vi "Merge Configs.vi"(7 "Dispose From Config (T)":bool=TRUE, 8 "error in (no error)":errorcluster, 9 "Merge Hierarchy (Root)":string[](array[string]), 10 "From Config":refnum<class "Config Manager.lvclass">, 11 "Config Manager in":refnum<class "Config Manager.lvclass">) -> (0 "error out":errorcluster, 3 "Config Manager out":refnum<class "Config Manager.lvclass">)   [LabVIEW 2023, in "CDM-Config.lvlib" / "Config Manager.lvclass"]
doc: "Merges the <b>From</b> Config into this Config. Any elements that are present in <b>From</b> and not in this config will be created, any values that are not blank in <b>From</b> will be written to this config, and Meta fields will be written to this config.\n\nBy default the <b>From</b> config will be cleaned up once the merge completes, leaving it unavailable for further use. To leave it available ensure setting <b>Dispose From Config</b> to False.\n\nOptionally a <b>Merge Hierarchy</b> can be specified and all elements in the <b>From</b> config will be merged in with the specified hierarchy element as the parent."
uses:
  Config Manager.lvclass
  Config Manager.lvclass/Config Manager.ctl
  Config Element/Write Variant Value.vi
  Config Element/Config Element.lvclass
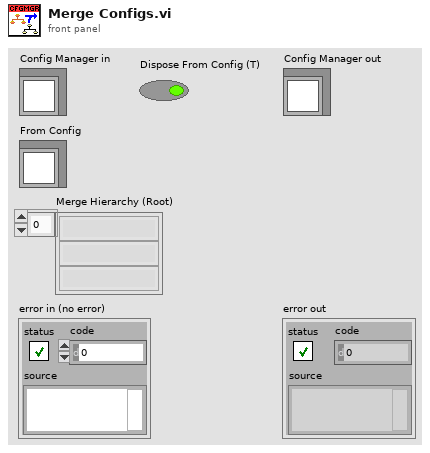
[diagram p1: front panel]
types:
  T1 = typedef "CDM-Config.lvlib/Config Manager.lvclass/Ref Data.ctl" = cluster{"Elements":refnum<class "Config Element.lvclass">[], "Hierarchy Map":map{string[], i32}, "Element Map":map{refnum<class "Config Element.lvclass">, i32}}
  T2 = typedef "CDM-Config.lvlib/Meta Data.ctl" = cluster{"Name":string, "Value":string}
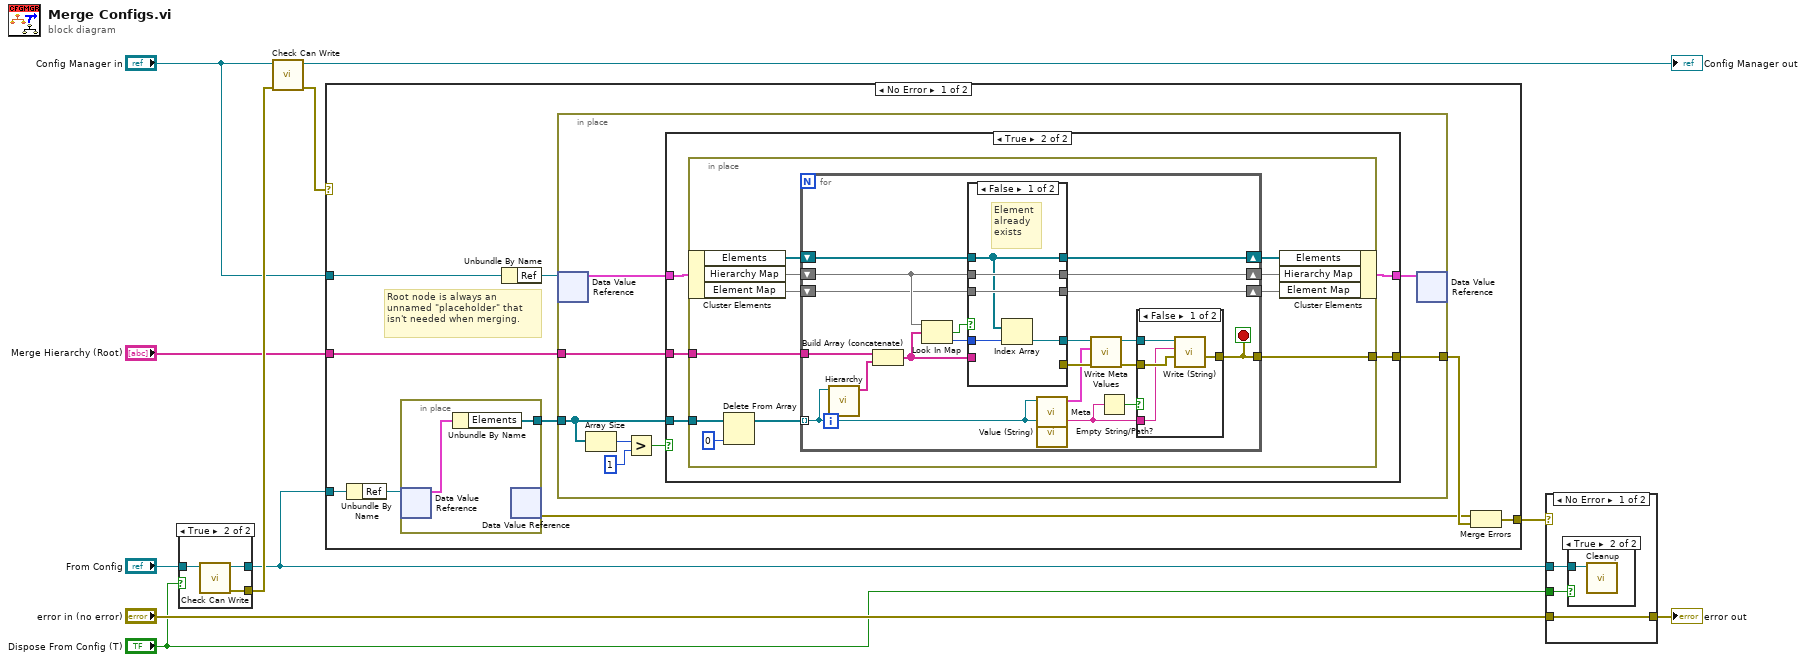
[diagram p0: block diagram]
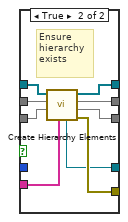
[diagram p3: hidden frame]
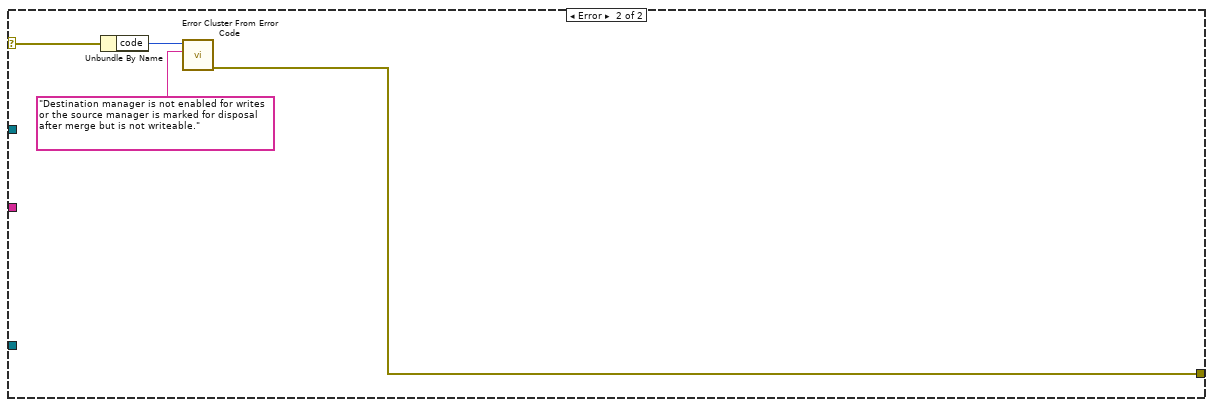
[diagram p5: hidden frame]
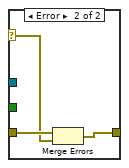
[diagram p8: hidden frame]
diagram:
  n1 = case shown="True" "Dispose From Config (T)" {
    tunnel: "From Config" -> [w12 w15]
    tunnel: [w12 w14] -> w5
    tunnel: [_ w13] -> w11
    frame False {
    }
    frame True {
      n2 = call "Check Can Write.vi"("Config Manager in"=w15) -> ("error out"=w13:errorcluster, "Config Manager out"=w14:refnum<class "Config Manager.lvclass">)  [unwired: 9 in]
    }
  }
  n3 = call "Check Can Write.vi"("error in (no error)"=w11, "Config Manager in"="Config Manager in") -> ("error out"=w1:errorcluster, "Config Manager out"=→"Config Manager out":refnum<class "Config Manager.lvclass">)  [unwired: 8 in]
  n4 = case shown="No Error" w1 {
    selector: w1 -> [_ w94]
    tunnel: [w23 w91] -> w9
    tunnel: "Merge Hierarchy (Root)" -> [w21 _]
    tunnel: w5 -> [w17 _]
    tunnel: "Config Manager in" -> [w16 _]
    frame No Error {
      # "Root node is always an unnamed \"placeholder\" that isn't needed when merging."
      n5 = Unbundle By Name(w17) -> ("Ref"=w20:refnum<data-value>)
      n6 = in-place {
        in-place-border: [w25] -> w19
        n7 = in-place-dvr #1(w20) -> (w26:T1)  [unwired: 1 out]
        n8 = Unbundle By Name(w26) -> ("Elements"=w25:refnum<class "Config Element.lvclass">[])
        n9 = in-place-dvr #1() -> (w18:errorcluster)  [unwired: 1 in, 1 out]
      }
      n10 = Unbundle By Name(w16) -> ("Ref"=w24:refnum<data-value>)
      n11 = in-place {
        in-place-border: [w29] -> w22
        in-place-border: w21 -> [w28]
        in-place-border: w19 -> [w27]
        n12 = in-place-dvr #2(w24) -> (w34:T1)  [unwired: 1 out]
        n13 = Array Size(array=w27) -> (size(s)=w33:i32)
        n14 = Greater?(x=w33, y=1) -> (0:w31:bool)
        n15 = case shown="True" w31 {
          tunnel: w34 -> [w35 w39]
          tunnel: w27 -> [_ w40]
          tunnel: [w35 w38] -> w30
          tunnel: [_ w37] -> w29
          tunnel: w28 -> [_ w36]
          frame False {
            # "From is empty (only has empty root node) so nothing to do."
          }
          frame True {
            n16 = in-place {
              in-place-border: w40 -> [w51]
              in-place-border: [w42] -> w37
              in-place-border: w36 -> [w41]
              n17 = in-place-cluster #3(w39) -> ("Elements"=w48:refnum<class "Config Element.lvclass">[], "Hierarchy Map"=w47:map{string[], i32}, "Element Map"=w46:map{refnum<class "Config Element.lvclass">, i32})
              n18 = Delete From Array(array=w51, index=0) -> (array with subset deleted=w49:refnum<class "Config Element.lvclass">[])  [unwired: 1 in, 1 out]
              n19 = for {
                tunnel: w49 -> [w56] mode=indexing
                shift-right: [w65] -> w43
                shift-left: w46 -> [w68]
                shift-right: [w63] -> w45
                shift-left: w48 -> [w70]
                shift-right: [w64] -> w44
                shift-left: w47 -> [w69]
                tunnel: [w52] -> w42
                tunnel: w41 -> [w60]
                stop <- w52 stop-if-true
                n20 = call "Hierarchy.vi"("Config Element in"=w56) -> ("Hierarchy"=w62:string[])  [unwired: 9 in, 1 out]
                n21 = Build Array (concatenate)(w60, w62) -> (w61:string[])
                n22 = Look In Map(map=w69, key=w61) -> (key not found?=w67:bool, value=w66:i32)  [unwired: 1 in]
                n23 = case shown="False" w67 {
                  tunnel: w70 -> [w73 w85]
                  tunnel: w69 -> [w74 w84]
                  tunnel: w68 -> [w75 w83]
                  tunnel: w66 -> [w76 _]
                  tunnel: [w75 w82] -> w65
                  tunnel: [w74 w81] -> w64
                  tunnel: [w73 w80] -> w63
                  tunnel: w61 -> [_ w79]
                  tunnel: [w72 w77] -> w57
                  tunnel: [_ w78] -> w71
                  frame False {
                    # "Element already exists"
                    n24 = Index Array(array=w73, index=w76) -> (element=w72:refnum<class "Config Element.lvclass">)
                  }
                  frame True {
                    # "Ensure hierarchy exists"
                    n25 = call "Create Hierarchy Elements.vi"("Hierarchy"=w79, "Element Map in"=w83, "Hierarchy Map in"=w84, "Elements in"=w85) -> ("error out"=w78:errorcluster, "Element Map"=w82:map{refnum<class "Config Element.lvclass">, i32}, "Hierarchy Map"=w81:map{string[], i32}, "Elements"=w80:refnum<class "Config Element.lvclass">[], "New Element"=w77:refnum<class "Config Element.lvclass">)  [unwired: 3 in]
                  }
                }
                n26 = call "Meta.vi"("Config Element in"=w56) -> ("Meta Data"=w55:T2[])  [unwired: 9 in, 1 out]
                n27 = call "Value (String).vi"("Config Element in"=w56) -> ("String Value"=w54:string)  [unwired: 9 in, 1 out]
                n28 = call "Write Meta Values.vi"("error in (no error)"=w71, "Meta Data"=w55, "Config Element in"=w57) -> ("error out"=w59:errorcluster, "Config Element out"=w58:refnum<class "Config Element.lvclass">)  [unwired: 7 in]
                n29 = Empty String/Path?(string/path=w54) -> (empty?=w53:bool)
                n30 = case shown="False" w53 {
                  tunnel: [w89 w90] -> w52
                  tunnel: w59 -> [w88 w90]
                  tunnel: w58 -> [w87 _]
                  tunnel: w54 -> [w86 _]
                  frame False {
                    n31 = call "Write (String).vi"("error in (no error)"=w88, "String Value"=w86, "Config Element in"=w87) -> ("error out"=w89:errorcluster)  [unwired: 7 in, 1 out]
                  }
                  frame True {
                  }
                }
              }
              n32 = in-place-cluster #3("Elements"=w45, "Hierarchy Map"=w44, "Element Map"=w43) -> (w38:T1)
            }
          }
        }
        n33 = in-place-dvr #2(w30) -> ()  [unwired: 2 out]
      }
      n34 = Merge Errors(w18, w22) -> (w23:errorcluster)
    }
    frame Error {
      n35 = Unbundle By Name(w94) -> ("code"=w93:i32)
      n36 = call <vilib>:"Error Cluster From Error Code.vi"("error message (\"\")"="Destination manager is not enabled for writes or the source manager is marked for disposal after merge but is not writeable." ("error message (\"\")"), "error code (0)"=w93) -> ("error out"=w91:errorcluster)  [unwired: 7 in]
    }
  }
  n37 = case shown="No Error" w9 {
    selector: w9 -> [_ w100]
    tunnel: w5 -> [w97 _]
    tunnel: "Dispose From Config (T)" -> [w96 _]
    tunnel: "error in (no error)" -> [w95 w101]
    tunnel: [w95 w99] -> w6
    frame No Error {
      n38 = case shown="True" w96 {
        tunnel: w97 -> [_ w98]
        frame False {
        }
        frame True {
          n39 = call "Cleanup.vi"("Config Manager in"=w98) -> ()  [unwired: 10 in, 1 out]
        }
      }
    }
    frame Error {
      n40 = Merge Errors(w101, w100) -> (w99:errorcluster)
    }
  }
  "error out" <- w6
